vi "GetKeyValue.vi"(5 "ConfigurationFilePath":path, 7 "Section":string, 9 "Key":string, 11 "error in":errorcluster) -> (6 "Value":string, 15 "error out":errorcluster)   [LabVIEW 2020, in "DMMFactory.lvlib" / "DMMFactory.lvclass"]
uses:
  DMMFactory.lvclass
  <vilib>/Utility/config.llb/Read Key (String).vi
  <vilib>/Utility/config.llb/NI_LVConfig.lvlib
panel:
  out "found?":bool
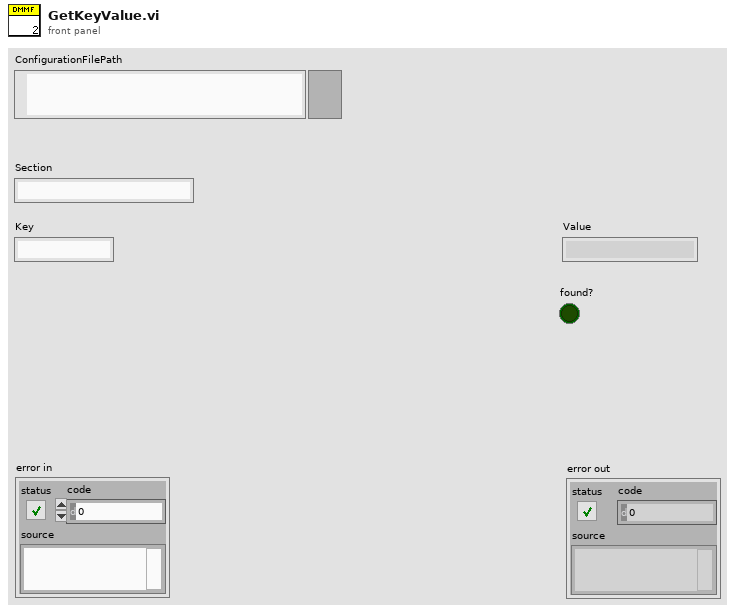
[diagram p1: front panel]
types:
  T1 = typedef "NI_LVConfig.lvlib/Config Data RefNum.ctl" = refnum<k1>
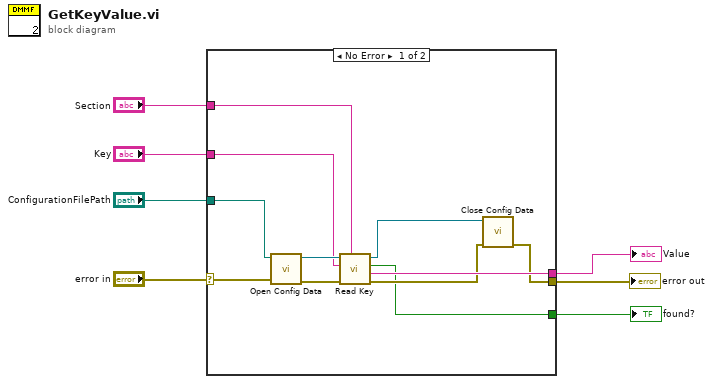
[diagram p0: block diagram]
diagram:
  n1 = case shown="No Error" "error in" {
    selector: "error in" -> [w18 w19]
    tunnel: "ConfigurationFilePath" -> [w17 _]
    tunnel: "Key" -> [w14 _]
    tunnel: "Section" -> [w13 _]
    tunnel: [w12 _] -> w3
    tunnel: [w10 w19] -> w2
    tunnel: [w8 _] -> w1
    frame No Error {
      n2 = call <vilib>:"Open Config Data.vi"("error in (no error)"=w18, "configuration file path"=w17) -> ("error out"=w16:errorcluster, "refnum"=w15:T1)  [unwired: 7 in, 1 out]
      n3 = call-poly <vilib>:"Read Key.vi"("section"=w13, "error in (no error)"=w16, "key"=w14, "refnum"=w15) -> ("error out"=w11:errorcluster, "value"=w12:string, "found?"=w8:bool, "refnum out"=w9:T1)  [unwired: 4 in]
      n4 = call <vilib>:"Close Config Data.vi"("error in (no error)"=w11, "refnum"=w9) -> ("error out"=w10:errorcluster)  [unwired: 8 in, 1 out]
    }
    frame Error {
    }
  }
  "error out" <- w2
  "Value" <- w3
  "found?" <- w1
